vi "Write Succeed State .vi"(8 "error in (no error)":errorcluster, 10 "Succeed State":T1, 11 "abs_Test Boolean in":refnum<class "abs_Test Boolean.lvclass">) -> (0 "error out":errorcluster, 3 "abs_Test Boolean out":refnum<class "abs_Test Boolean.lvclass">)   [LabVIEW 2021, in "BT.lvlib" / "abs_Test Boolean.lvclass"]
uses:
  abs_Test Boolean.lvclass
  Support/Succeed State.ctl
  abs_Test Boolean.lvclass/abs_Test Boolean.ctl
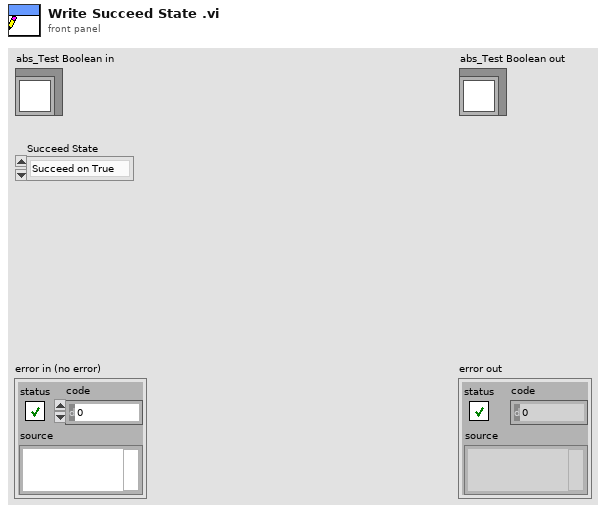
[diagram p1: front panel]
types:
  T1 = typedef "BT.lvlib/abs_Test Boolean.lvclass/Succeed State.ctl" = enum16{"Succeed on True", "Succeed on Fail"}
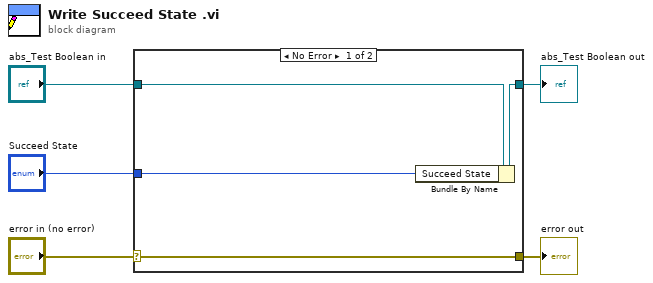
[diagram p0: block diagram]
diagram:
  n1 = case shown="No Error" "error in (no error)" {
    selector: "error in (no error)" -> [w9 w10]
    tunnel: [w9 w10] -> w4
    tunnel: [w7 w11] -> w2
    tunnel: "abs_Test Boolean in" -> [w8 w11]
    tunnel: "Succeed State" -> [w6 _]
    frame No Error {
      n2 = Bundle By Name(cluster=w8, "Succeed State"=w6) -> (w7:refnum<class "abs_Test Boolean.lvclass">)
    }
    frame Error {
    }
  }
  "error out" <- w4
  "abs_Test Boolean out" <- w2
